vi "PID_feedback_pel.vi"(4 "Reintialize":bool[](array[boolean]), 5 "currentT":dbl[](array[numeric]), 6 "dt (s)":dbl=-1.0 format="%.3f", 7 "LimitLogicIn":bool[](array[boolean]), 9 "SetTension":dbl[](array[numeric]), 10 "PID_OP_Lim":cluster{"output high":dbl, "output low":dbl}[](array[cluster])=[{"output high"=100.0, "output low"=-100.0}] {"output low" format="%.2f"; "output high" format="%.2f"}, 11 "Constants LL":T1) -> (1 "pidOP":dbl[](array[numeric]), 3 "limit logic out":bool[](array[boolean]))   [LabVIEW 2017]
uses:
  typeDef/constants_LL.ctl
  <vilib>/addons/control/pid/pid.llb/PID Advanced (DBL Array).vi
  <vilib>/addons/control/pid/pid.llb/PID Parameter Manager (DBL Array).vi
  <vilib>/addons/control/pid/pid.llb/PID Derivative Action Buffered (DBL Array).vi
  <vilib>/addons/control/pid/pid.llb/PID Get Advanced Error (DBL Array).vi
  <vilib>/addons/control/pid/pid.llb/PID Integral Action Buffered (DBL Array).vi
  <vilib>/addons/control/pid/pid.llb/PID Resize 1D Array.vi
  <vilib>/addons/control/pid/pid.llb/PID Get Advanced Error (DBL).vi
  <vilib>/addons/control/pid/NI_PID_pid.lvlib
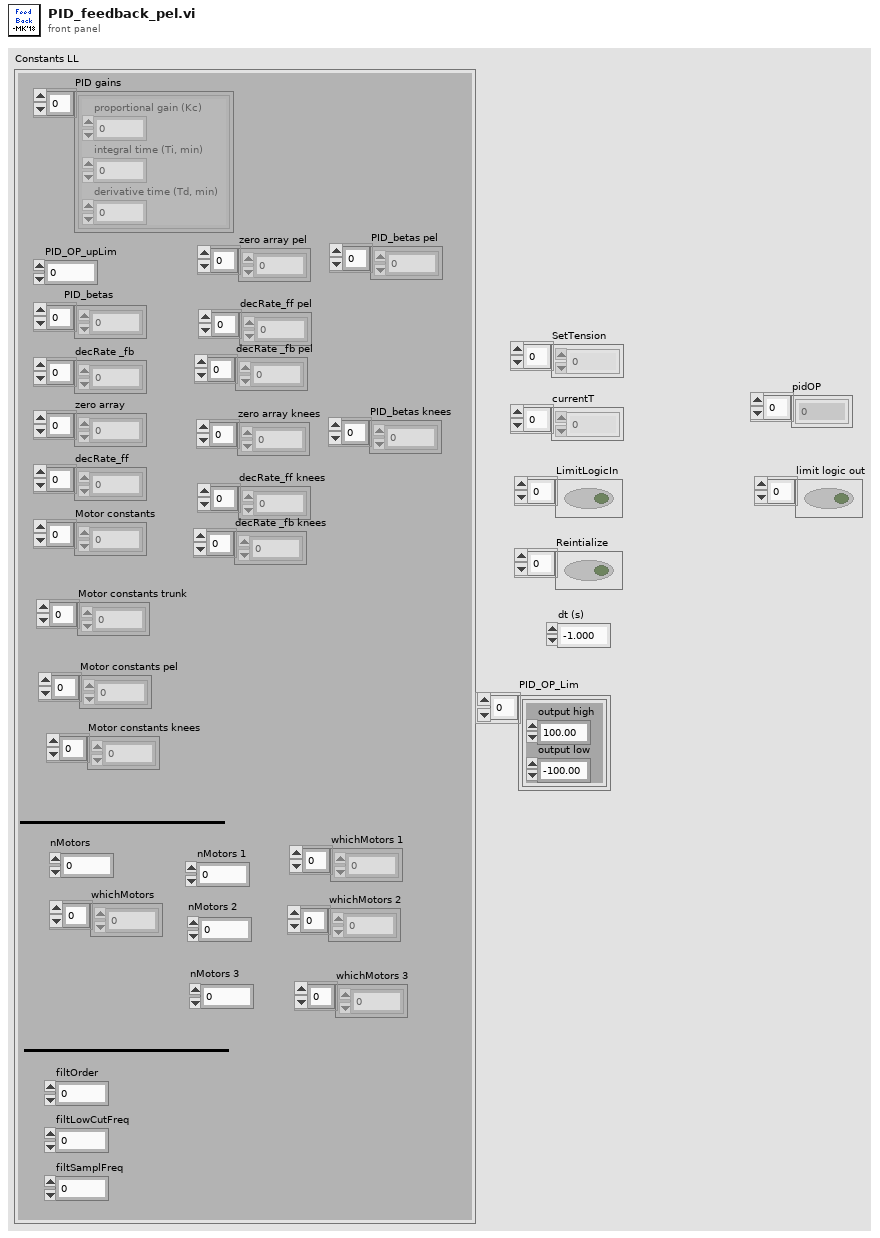
[diagram p1: front panel]
types:
  T1 = typedef "constants_LL.ctl" = cluster{"zero array":dbl[], "decRate_ff":dbl[], "Motor constants":dbl[], "PID gains":cluster{"proportional gain (Kc)":dbl, "integral time (Ti, min)":dbl, "derivative time (Td, min)":dbl}[], "decRate _fb":dbl[], "PID_OP_upLim":dbl, "nMotors":i32, "PID_betas":dbl[], "filtOrder":i32, "filtLowCutFreq":dbl, "filtSamplFreq":dbl, "whichMotors":i32[], "nMotors 1":i32, "nMotors 2":i32, "Motor constants pel":dbl[], "Motor constants trunk":dbl[], "whichMotors 1":i32[], "whichMotors 2":i32[], "zero array pel":dbl[], "decRate_ff pel":dbl[], "decRate _fb pel":dbl[], "PID_betas pel":dbl[], "whichMotors 3":i32[], "nMotors 3":i32, "Motor constants knees":dbl[], "zero array knees":dbl[], "decRate_ff knees":dbl[], "decRate _fb knees":dbl[], "PID_betas knees":dbl[]}
  T2 = cluster{"proportional gain (Kc)":dbl, "integral time (Ti, min)":dbl, "derivative time (Td, min)":dbl}[]
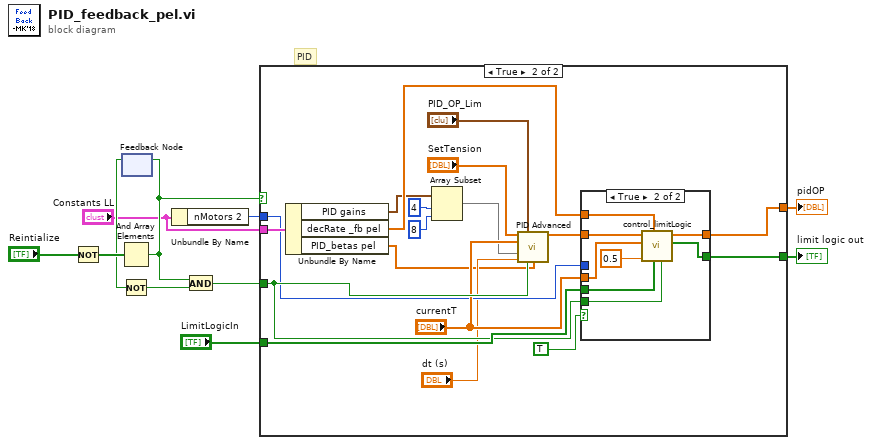
[diagram p0: block diagram]
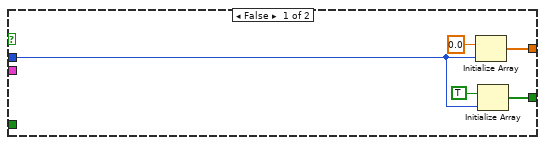
[diagram p2: hidden frame]
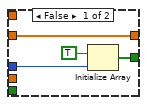
[diagram p3: hidden frame]
diagram:
  # "PID"
  n1 = Not(x="Reintialize") -> (.not. x?=w7:bool[])
  n2 = And Array Elements(Boolean array=w7) -> (logical AND=w9:bool)
  n3 = feedback #1() -> (w4:bool)  [unwired: 1 in]
  n4 = Not(x=w4) -> (.not. x?=w3:bool)
  n5 = feedback-in #1(w9) -> ()
  n6 = Unbundle By Name("Constants LL") -> ("nMotors 2"=w1:i32)
  n7 = And(x=w9, y=w3) -> (x .and. y?=w6:bool)
  n8 = case shown="True" w9 {
    tunnel: [w15 w17] -> w5
    tunnel: w6 -> [_ w32]
    tunnel: "LimitLogicIn" -> [_ w34]
    tunnel: [w13 w33] -> w11
    tunnel: w1 -> [w12 w29]
    tunnel: "Constants LL" -> [_ w30]
    frame False {
      n9 = Initialize Array(0.0 ("element"), w12) -> (w15:dbl[])
      n10 = Initialize Array(TRUE, w12) -> (w13:bool[])
    }
    frame True {
      n11 = Unbundle By Name(w30) -> ("PID gains"=w21:T2, "decRate _fb pel"=w27:dbl[], "PID_betas pel"=w26:dbl[])
      n12 = Array Subset(array=w21, index=4, length=8) -> (w20:T2)
      n13 = call-poly <vilib>:"PID Advanced.vi"("setpoint"="SetTension", "output range"="PID_OP_Lim", "process variable"="currentT", "PID gains"=w20, "dt (s)"="dt (s)", "reinitialize? (F)"=w32, "beta"=w26) -> ("output"=w18:dbl[])  [unwired: 7 in, 1 out]
      n14 = case shown="True" TRUE {
        tunnel: w32 -> [_ w46]
        tunnel: w34 -> [_ w45]
        tunnel: [w36 w44] -> w33
        tunnel: w27 -> [_ w43]
        tunnel: w18 -> [w38 w42]
        tunnel: [w38 w41] -> w17
        tunnel: "currentT" -> [_ w40]
        tunnel: w29 -> [w35 _]
        frame False {
          n15 = Initialize Array(TRUE, w35) -> (w36:bool[])
        }
        frame True {
          n16 = call "control_limitLogic.vi"("reinitialize"=w46, "limit logic in"=w45, "dec rate"=w43, "diff"=0.5 ("y"), "Initial op"=w40, "Input"=w42) -> ("limit logic out"=w44:bool[], "output"=w41:dbl[])  [unwired: 4 in]
        }
      }
    }
  }
  "limit logic out" <- w11
  "pidOP" <- w5
